vi "FindBillardBox.vi"(8 "error in (no error)":errorcluster, 10 "Dark Blue Frame":T2={"Rmin"=0.0, " Rmax"=24.0, "Gmin"=0.0, "Gmax"=49.0, "Bmin"=100.0, "Bmax"=119.0}, 11 "Path":path) -> (0 "error out":errorcluster, 2 "Billard Box":T1)   [LabVIEW 2025]
doc: "Déterminer automatiquement la boite englobante du cadre bleu foncé du billard afin d'obtenir les\nlimites Xmin, Xmax, Ymin, Ymax. Ce rectangle (Billard Box) est ensuite utilisé pour la recherche des boules dans le programme C."
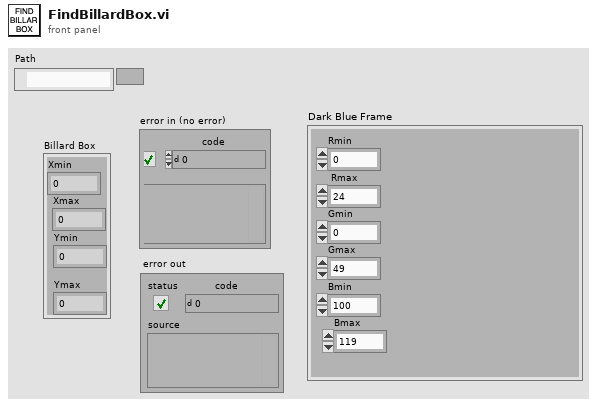
[diagram p1: front panel]
types:
  T1 = cluster{"Xmin":dbl, "Xmax":dbl, "Ymin":dbl, "Ymax":dbl}
  T2 = cluster{"Rmin":dbl, " Rmax":dbl, "Gmin":dbl, "Gmax":dbl, "Bmin":dbl, "Bmax":dbl}
  T3 = typedef "imagedata.ctl" = cluster{"image type":i32, "image depth":i32, "image":u8[], "mask":u8[], "colors":u32[], "Rectangle":cluster{"left":i16, "top":i16, "right":i16, "bottom":i16}}
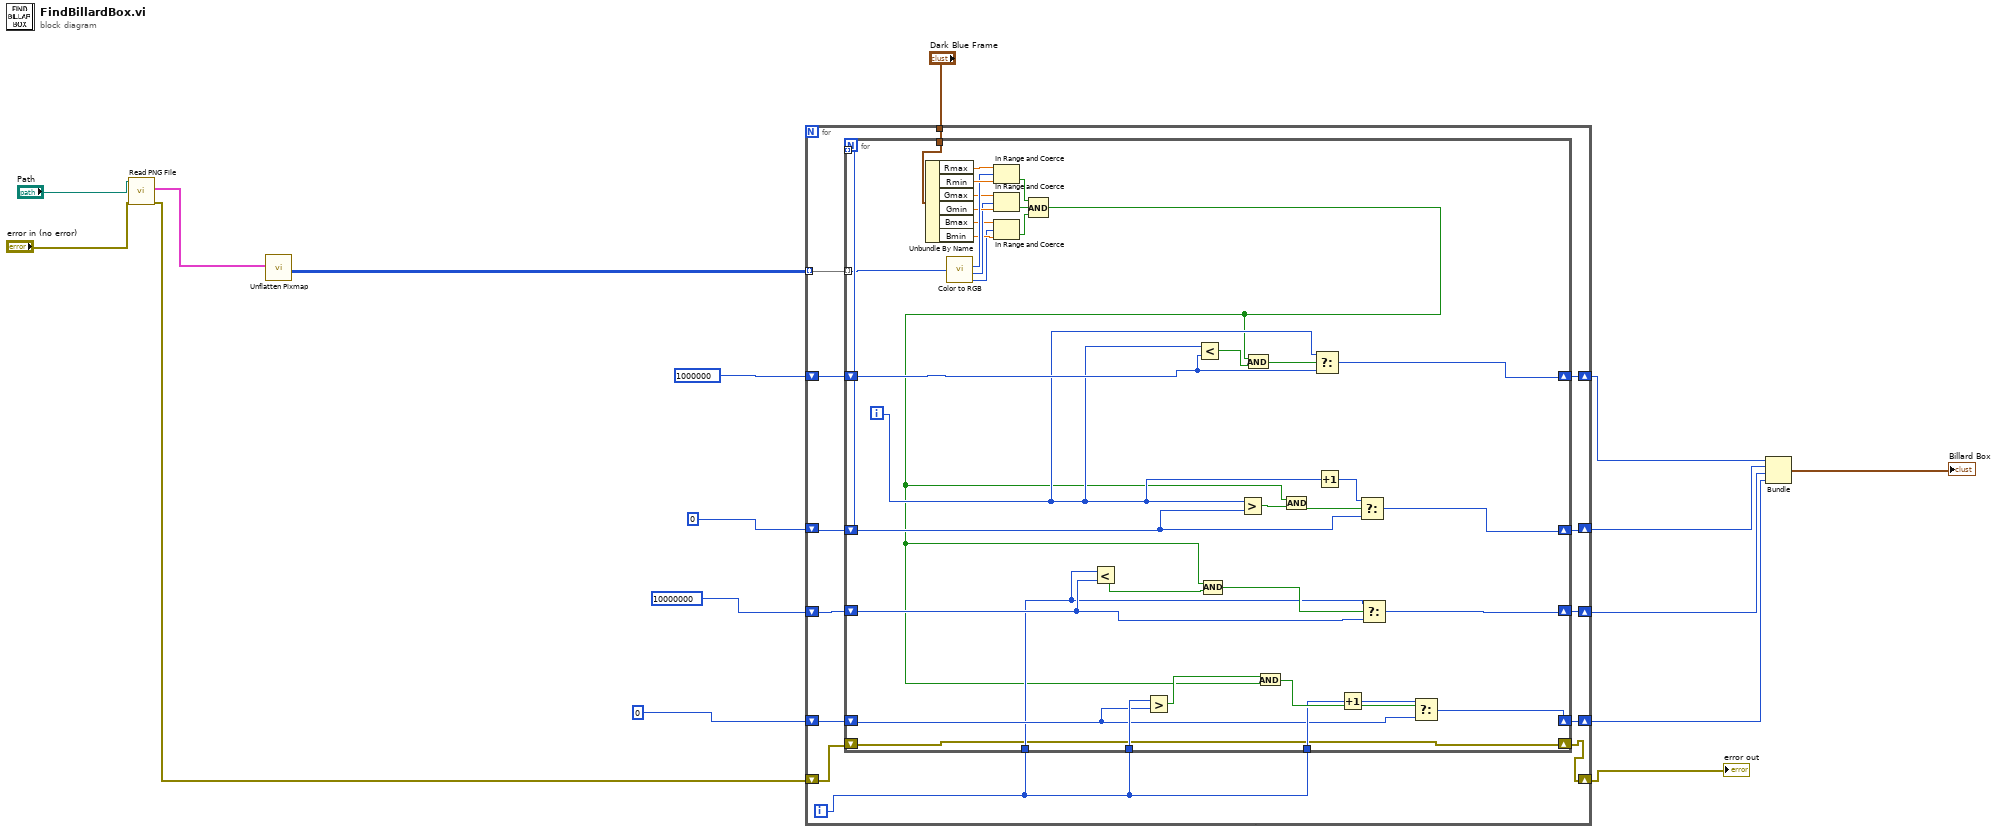
[diagram p0: block diagram]
diagram:
  # "."
  n1 = call <vilib>:"Read PNG File.vi"("error in (no error)"="error in (no error)", "path to PNG file"="Path") -> ("error out"=w9:errorcluster, "image data"=w8:T3)  [unwired: 7 in, 1 out]
  n2 = call <vilib>:"Unflatten Pixmap.vi"("image data"=w8) -> ("24-bit pixmap"=w7:u32[][])  [unwired: 4 in, 6 out]
  n3 = for {
    tunnel: "Dark Blue Frame" -> [w29]
    tunnel: w7 -> [w23] mode=indexing
    shift-right: [w21] -> w3
    shift-left: 0 -> [w26]
    shift-right: [w18] -> w2
    shift-left: u32 10000000 -> [w24]
    shift-right: [w20] -> w4
    shift-left: 0 -> [w27]
    shift-right: [w19] -> w5
    shift-left: 1000000 -> [w28]
    shift-right: [w17] -> w1
    shift-left: w9 -> [w25]
    i -> [w22]
    n4 = for {
      shift-right: [w49] -> w20
      shift-left: w27 -> [w43]
      shift-right: [w52] -> w19
      shift-left: w28 -> [w51]
      shift-right: [w46] -> w18
      shift-left: w24 -> [w44]
      shift-right: [w45] -> w21
      shift-left: w26 -> [w35]
      tunnel: w29 -> [w67]
      tunnel: [w43] -> _ mode=indexing
      tunnel: w23 -> [w41] mode=indexing
      tunnel: w22 -> [w36]
      tunnel: w22 -> [w37]
      tunnel: w22 -> [w34]
      shift-right: [w30] -> w17
      shift-left: w25 -> [w30]
      i -> [w32]
      n5 = Unbundle By Name(w67) -> ("Rmax"=w66:dbl, "Rmin"=w65:dbl, "Gmax"=w63:dbl, "Gmin"=w62:dbl, "Bmax"=w60:dbl, "Bmin"=w59:dbl)
      n6 = call <vilib>:"Color to RGB.vi"("Color"=w41) -> ("R"=w64:u8, "G"=w61:u8, "B"=w58:u8)  [unwired: 1 out]
      n7 = In Range and Coerce(upper limit=w66, x=w64, lower limit=w65) -> (In Range?=w57:bool)  [unwired: 1 out]
      n8 = In Range and Coerce(upper limit=w63, x=w61, lower limit=w62) -> (In Range?=w56:bool)  [unwired: 1 out]
      n9 = In Range and Coerce(upper limit=w60, x=w58, lower limit=w59) -> (In Range?=w55:bool)  [unwired: 1 out]
      n10 = Compound Arithmetic op=AND(w57, w56, w55) -> (w31:bool)
      n11 = Less?(x=w34, y=w44) -> (x < y?=w48:bool)
      n12 = Greater?(x=w36, y=w35) -> (0:w40:bool)
      n13 = Less?(x=w32, y=w51) -> (x < y?=w54:bool)
      n14 = Compound Arithmetic op=AND(w31, w48) -> (w47:bool)
      n15 = Greater?(x=w32, y=w43) -> (0:w42:bool)
      n16 = Compound Arithmetic op=AND(w31, w54) -> (w53:bool)
      n17 = And(x=w40, y=w31) -> (x .and. y?=w39:bool)
      n18 = Compound Arithmetic op=AND(w31, w42) -> (w50:bool)
      n19 = Select(t=w32, s=w53, f=w51) -> (s? t:f=w52:i32)
      n20 = Increment(x=w32) -> (x+1=w33:i32)
      n21 = Increment(x=w37) -> (x+1=w38:i32)
      n22 = Select(t=w33, s=w50, f=w43) -> (s? t:f=w49:i32)
      n23 = Select(t=w34, s=w47, f=w44) -> (s? t:f=w46:u32)
      n24 = Select(t=w38, s=w39, f=w35) -> (s? t:f=w45:i32)
    }
  }
  "error out" <- w1
  n25 = Bundle(w5, w4, w2, w3) -> (→"Billard Box":cluster{i32, i32, u32, i32})  [unwired: 1 in]
